vi "Agilent E4980 Read Measurement.vi"() -> ()   [LabVIEW 2019]
doc: "This example shows how to configure a measurement and take readings."
uses:
  Agilent E4980.lvlib
panel:
  in  "Averaging Factor (1)":i32=1
  in  "Measurement Time (1: Medium)":u16(ring)=1 items=["Short", "Medium", "Long"]
  in  "Signal Level (1.0 V)":dbl=1.0
  in  "Signal Type (0: Voltage)":u16(ring) items=["Voltage", "Current"]
  in  "Signal Frequency (1000 Hz)":dbl=1000.0
  in  "Enable Auto Range (T:Enable)":bool=TRUE
  in  "Manual Impedance Range (3: 100 Ohms)":i32(ring)=3 items=["100m", "1", "10", "100", "300", "1K", "3K", "10K", "30K", "100K"]
  in  "Function (0: Cp-D)":u16(ring) items=["Cp-D", "Cp-Q", "Cp-G", "Cp-Rp", "Cs-D", "Cs-Q", "Cs-Rs", "Lp-D", "Lp-Q", "Lp-G", "Lp-Rp", "Lp-Rdc", "Ls-D", "Ls-Q", "Ls-Rs", "Ls-Rdc", "R-X", "Z-thd", "Z-thr", "G-B", "Y-thd", "Y-thr", "Vdc-Idc"]
  out "Primary Parameter":dbl
  out "Secondary Parameter":dbl
  in  "VISA resource name":refnum<visa-resource-name>
  # "(c) 2007-2015 National Instruments.  ALL RIGHTS RESERVED."
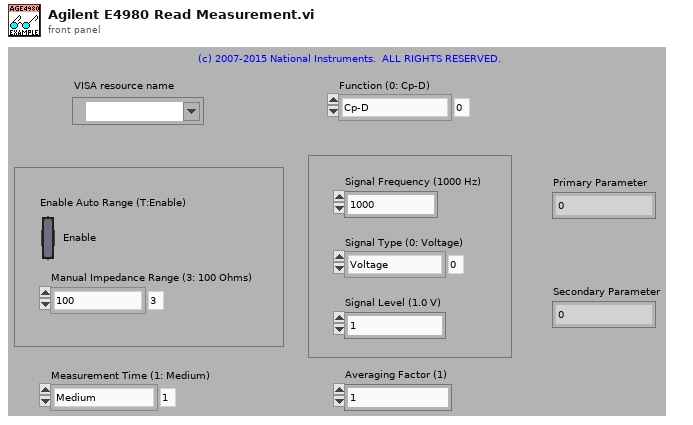
[diagram p1: front panel]
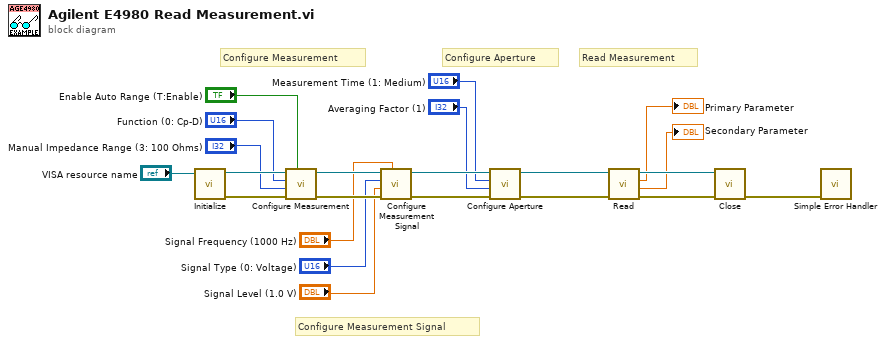
[diagram p0: block diagram]
diagram:
  # "Configure Aperture"
  # "Configure Measurement Signal"
  # "Read Measurement"
  # "Configure Measurement"
  n1 = call "Initialize.vi"("VISA resource name"="VISA resource name") -> ("error out"=w20:errorcluster, "VISA resource name out"=w21:refnum<visa-resource-name>)  [unwired: 9 in]
  n2 = call "Configure Measurement.vi"("Enable Auto Range (T:Enable)"="Enable Auto Range (T:Enable)", "error in (no error)"=w20, "Manual Impedance Range (3: 100 Ohms)"="Manual Impedance Range (3: 100 Ohms)", "Function (0: Cp-D)"="Function (0: Cp-D)", "VISA resource name"=w21) -> ("error out"=w13:errorcluster, "VISA resource name out"=w14:refnum<visa-resource-name>)  [unwired: 5 in]
  n3 = call "Configure Measurement Signal.vi"("Signal Frequency (1000 Hz)"="Signal Frequency (1000 Hz)", "error in (no error)"=w13, "Signal Level (1.0 V)"="Signal Level (1.0 V)", "Signal Type (0: Voltage)"="Signal Type (0: Voltage)", "VISA resource name"=w14) -> ("error out"=w11:errorcluster, "VISA resource name out"=w12:refnum<visa-resource-name>)  [unwired: 5 in]
  n4 = call "Configure Aperture.vi"("error in (no error)"=w11, "Averaging Factor (1)"="Averaging Factor (1)", "Measurement Time (1: Medium)"="Measurement Time (1: Medium)", "VISA resource name"=w12) -> ("error out"=w9:errorcluster, "VISA resource name out"=w10:refnum<visa-resource-name>)  [unwired: 6 in]
  n5 = call "Read.vi"("error in (no error)"=w9, "VISA resource name"=w10) -> ("error out"=w18:errorcluster, "Secondary Parameter"=→"Secondary Parameter":dbl, "Primary Parameter"=→"Primary Parameter":dbl, "VISA resource name out"=w19:refnum<visa-resource-name>)  [unwired: 6 in]
  n6 = call "Close.vi"("error in (no error)"=w18, "VISA resource name"=w19) -> ("error out"=w15:errorcluster)  [unwired: 9 in]
  n7 = call <vilib>:"Simple Error Handler.vi"("error in (no error)"=w15) -> ()  [unwired: 4 in, 5 out]
